vi "Alternate BG Color.vi"(7 "Number of Rows":i32, 8 "错误输入":errorcluster, 9 "Second BG Color":u32(colorbox), 10 "First BG Color":u32(colorbox), 11 "Listbox Ref":refnum<vi>) -> (0 "错误输出":errorcluster, 3 "Dup Listbox Ref":refnum<vi>)   [LabVIEW 2012, in "Listbox Tool.lvlib"]
uses:
  Listbox Tool.lvlib
  Custom Type/Read and Write Mode.ctl
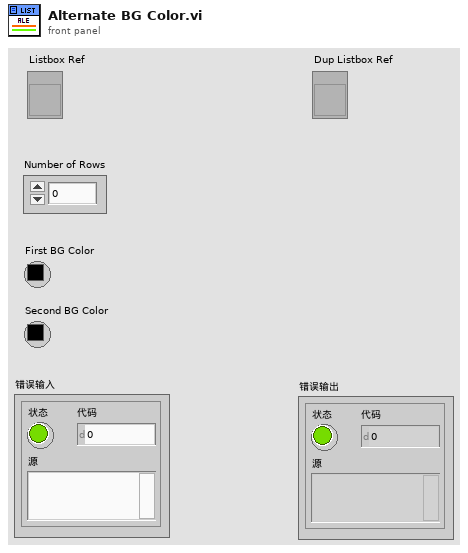
[diagram p1: front panel]
types:
  T1 = typedef "Listbox Tool.lvlib/Read and Write Mode.ctl" = enum16{"Read", "Write"}
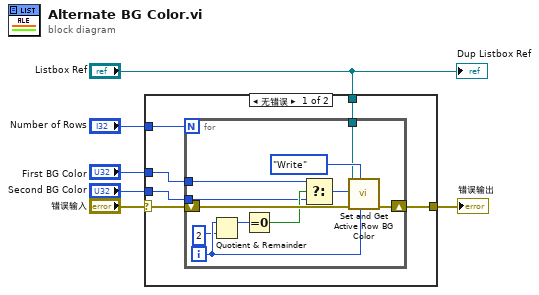
[diagram p0: block diagram]
diagram:
  n1 = case shown="无错误" "错误输入" {
    selector: "错误输入" -> [w12 w24]
    tunnel: [w11 w24] -> w5
    tunnel: "Number of Rows" -> [w10 _]
    tunnel: "First BG Color" -> [w9 _]
    tunnel: "Second BG Color" -> [w8 _]
    tunnel: "Listbox Ref" -> [w7 _]
    frame No Error {
      n2 = for {
        N: w10 -> [_]
        shift-right: [w21] -> w11
        shift-left: w12 -> [w22]
        tunnel: w9 -> [w16]
        tunnel: w8 -> [w15]
        tunnel: w7 -> [w13]
        i -> [w20]
        n3 = Quotient & Remainder(x=w20, y=2) -> (x-y*floor(x/y)=w18:i32)  [unwired: 1 out]
        n4 = Equal To 0?(x=w18) -> (x = 0?=w17:bool)
        n5 = Select(t=w16, s=w17, f=w15) -> (s? t:f=w14:u32)
        n6 = call "Set and Get Active Row BG Color.vi"("Active Row"=w20, "Mode"=Read_and_Write_Mode."Write", "错误输入"=w22, "CellBG In"=w14, "Listbox Ref"=w13) -> ("错误输出"=w21:errorcluster)  [unwired: 4 in, 2 out]
      }
    }
    frame Error {
    }
  }
  "错误输出" <- w5
  "Dup Listbox Ref" <- "Listbox Ref"
